vi "act_4-conv_C_F.vi"() -> ()   [LabVIEW 2010]
panel:
  out "deg F":dbl
  in  "deg C":dbl
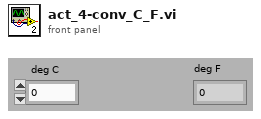
[diagram p1: front panel]
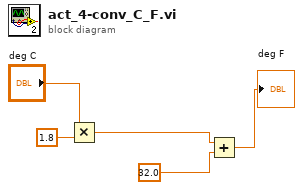
[diagram p0: block diagram]
diagram:
  n1 = Multiply(x="deg C", y=1.8) -> (x*y=w3:dbl)
  n2 = Add(x=w3, y=32.0) -> (x+y=→"deg F":dbl)
